vi "fi-destructor.vi"(8 "error in (no error)":errorcluster, 11 "frameInput in":refnum<class "bFrameIO.lvclass">) -> (0 "error out":errorcluster, 3 "frameInput out":refnum<class "bFrameIO.lvclass">)   [LabVIEW 2015, in "bFrameIO.lvclass"]
uses:
  bFrameIO.lvclass
  bFrameIO.lvclass/bFrameIO.ctl
  class.can.table/bAPPdata.lvclass
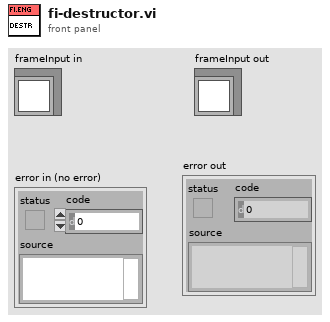
[diagram p1: front panel]
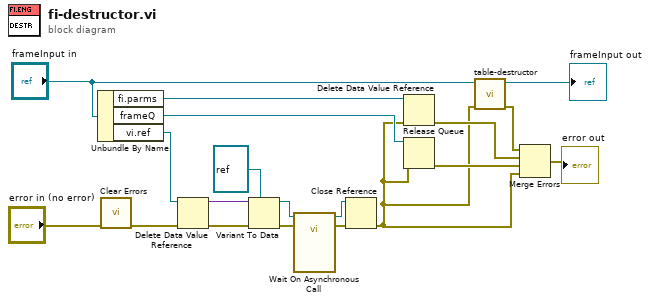
[diagram p0: block diagram]
diagram:
  n1 = Unbundle By Name("frameInput in") -> ("fi.parms"=w15:refnum<data-value>, "frameQ"=w17:refnum<queue>, "vi.ref"=w9:refnum<data-value>)
  n2 = call <vilib>:"Clear Errors.vi"("error in (no error)"="error in (no error)") -> ("error out"=w12:errorcluster)  [unwired: 5 in, 1 out]
  n3 = Delete Data Value Reference(data value reference=w9, error in=w12) -> (data value=w7:variant, error out=w10:errorcluster)
  n4 = Variant To Data(error in=w10, type=refnum<vi> refnum ("vi reference"), Variant=w7) -> (data=w5:refnum<vi>, error out=w8:errorcluster)
  n5 = call-by-ref "Wait On Asynchronous Call"(reference=w5, error in=w8) -> (reference out=w4:refnum<vi>, error out=w11:errorcluster)  [unwired: 10 in, 2 out]
  n6 = Close Reference(reference=w4, error in (no error)=w11) -> (error out=w1:errorcluster)
  n7 = Delete Data Value Reference(data value reference=w15, error in=w1) -> (error out=w14:errorcluster)  [unwired: 1 out]
  n8 = Release Queue(queue=w17, error in (no error)=w1) -> (error out=w16:errorcluster)  [unwired: 1 in, 2 out]
  n9 = call "table-destructor.vi"("error in (no error)"=w1, "CANtable in"="frameInput in") -> ("error out"=w2:errorcluster, "CANtable out"=→"frameInput out":refnum<class "bFrameIO.lvclass">)  [unwired: 8 in]
  n10 = Merge Errors(w2, w14, w16, w1) -> (→"error out":errorcluster)
